vi "niScope Create Configuration List.vi"(0 "instrument handle":refnum<k15>, 1 "set as active list":bool=TRUE, 5 "list name":string, 7 "step attributes":T1(array[ring])=[enum."Step Timer Time"], 11 "error in":errorcluster) -> (4 "instrument handle out":refnum<k15>, 15 "error out":errorcluster)   [LabVIEW 2013]
doc: "Use this function to create a Configuration List and to declare what attributes are in the Configuration List. Set the setAsActiveList parameter to make this list the active one."
uses:
  niScope_32.dll
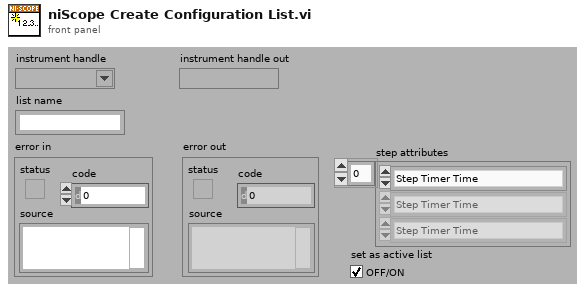
[diagram p1: front panel]
types:
  T1 = enum16{"Digital Gain", "Center frequency", "Phase I", "Phase Q", "Step Timer Time", "Bandpass Filter Enabled", "Configuration Time", "Equalization Coefficients", "Dither Enabled", "Trigger Level", "Trigger Hysteresis"}[]
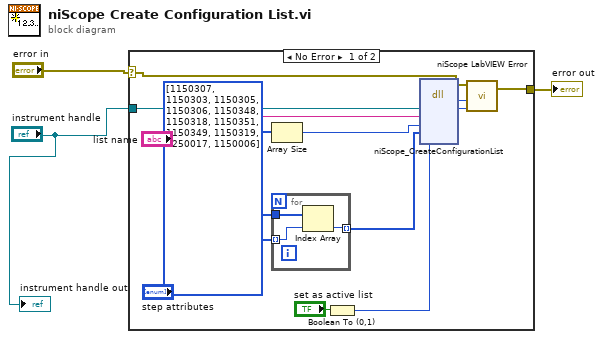
[diagram p0: block diagram]
diagram:
  n1 = case shown="No Error" "error in" {
    selector: "error in" -> [w10 w19]
    tunnel: [w11 w19] -> w2
    tunnel: "instrument handle" -> [w14 _]
    frame No Error {
      n2 = Array Size(array="step attributes") -> (size(s)=w9:i32)
      n3 = for {
        tunnel: "step attributes" -> [w18] mode=indexing
        tunnel: i32[] [1150307, 1150303, 1150305, 1150306, 1150348, 1150318, 1150351, 1150349, 1150319, 1250017, 1150006] -> [w17]
        tunnel: [w16] -> w4 mode=indexing
        n4 = Index Array(array=w17, index=w18) -> (element=w16:i32)
      }
      n5 = Boolean To (0,1)(Boolean="set as active list") -> (0, 1=w7:i16)
      n6 = dll-call lib="niScope_*.*" fn="niScope_CreateConfigurationList"("instrument handle"=w14, "listName"="list name", "bufferSize"=w9, "stepAttributes"=w4, "setAsActiveList"=w7) -> ("status"=w13:i32, "instrument handle"=w12:u32)  [unwired: 5 in, 4 out]
      n7 = call <instrlib>:"niScope LabVIEW Error.vi"("instrument handle"=w12, "niScope error code (0)"=w13, "error in (no error)"=w10) -> ("error out"=w11:errorcluster)  [unwired: 2 out]
    }
    frame Error {
    }
  }
  "error out" <- w2
  "instrument handle out" <- "instrument handle"
